vi "gen_logic_vi_with_cmd_array.vi"(9 "CmdInfo":T1, 10 "VI Paths":path) -> (2 "VI Paths Out":path=path "d:/Program Files (x86)/National Instruments/LabVIEW 2011/instr.lib/Agilent MXA Series/express/Utility/auto_gen_logic.vi")   [LabVIEW 2018]
uses:
  command_spec.ctl
  StudioHelper/Gtor/Mth/GenVI/Intf/GenStdVI/Mth/GenOneStdVI/TypeDefinitions/single_vi_spec.ctl
  StudioHelper/Gtor/Mth/GenVI/Intf/GenStdVI/Mth/GenOneStdVI/TypeDefinitions/single_cmd_spec.ctl
  StudioHelper/Gtor/Mth/GenVI/Intf/GenStdVI/Mth/GenOneStdVI/TypeDefinitions/single_control_spec.ctl
  StudioHelper/Gtor/Mth/GenVI/Intf/GenStdVI/Mth/GenOneStdVI/TypeDefinitions/control_data_type.ctl
  StudioHelper/Gtor/Mth/GenVI/Intf/GenStdVI/Mth/GenOneStdVI/TypeDefinitions/control_class.ctl
  StudioHelper/Gtor/Mth/GenVI/Intf/GenStdVI/Mth/GenOneStdVI/TypeDefinitions/ring_string_and_value.ctl
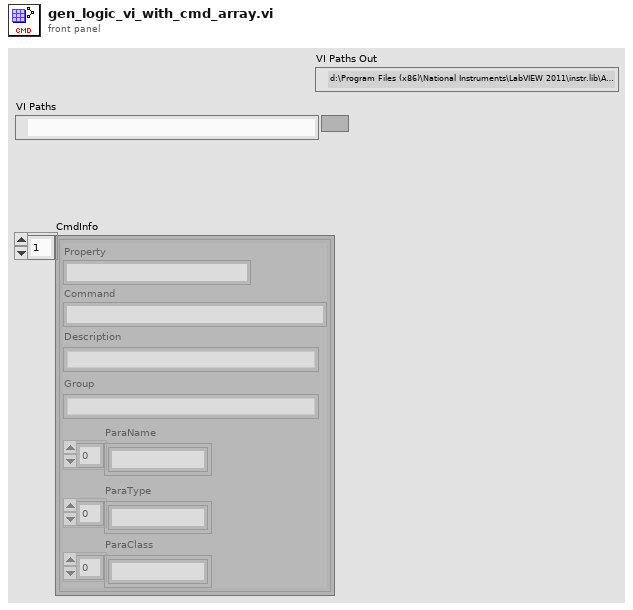
[diagram p1: front panel]
types:
  T1 = typedef "command_spec.ctl" = cluster{"Property":string, "Command":string, "Description":string, "Group":string, "ParaName":string[], "ParaType":string[], "ParaClass":string[]}[]
  T2 = typedef "single_vi_spec.ctl" = cluster{"Configure Specs In":T3[], "VI Paths":path, "Control Label Sequences":string[]}
  T3 = typedef "single_cmd_spec.ctl" = cluster{"Instrument Command":string, "Controls Specs":T4[]}
  T4 = typedef "single_control_spec.ctl" = cluster{"Control Label":string, "Control Data Type":T5, "Control Class":T6, "BD Text":string, "Ring Strings and Values":T7[], "Required Input":bool, "Default Value":string}
  T5 = typedef "control_data_type.ctl" = enum16{"DBL", "I32", "Boolean", "String", "U16", "U32", "EXT", "SGL", "I16", "U8", "I8", "I64", "U64", "Waveform", "Reference", "Variant", "Cluster"}
  T6 = typedef "control_class.ctl" = enum16{"Numeric", "Vertical Slide Switch", "Text Ring", "String", "Array", "VISAName", "WaveformGraph", "Cluster"}
  T7 = typedef "ring_string_and_value.ctl" = cluster{"String":string, "Value":dbl}
  T8 = typedef "auto_extracted_control_specs.ctl" = T9[]
  T9 = typedef "auto_extracted_control_spec.ctl" = cluster{"Control Data Type":T5, "Ring Text":string[], "Control Label":string, "Command Start Offset":i32, "Command Stop Offset":i32, "Control Class":T6, "Default Value":string, "Ring Strings and Values":T7[]}
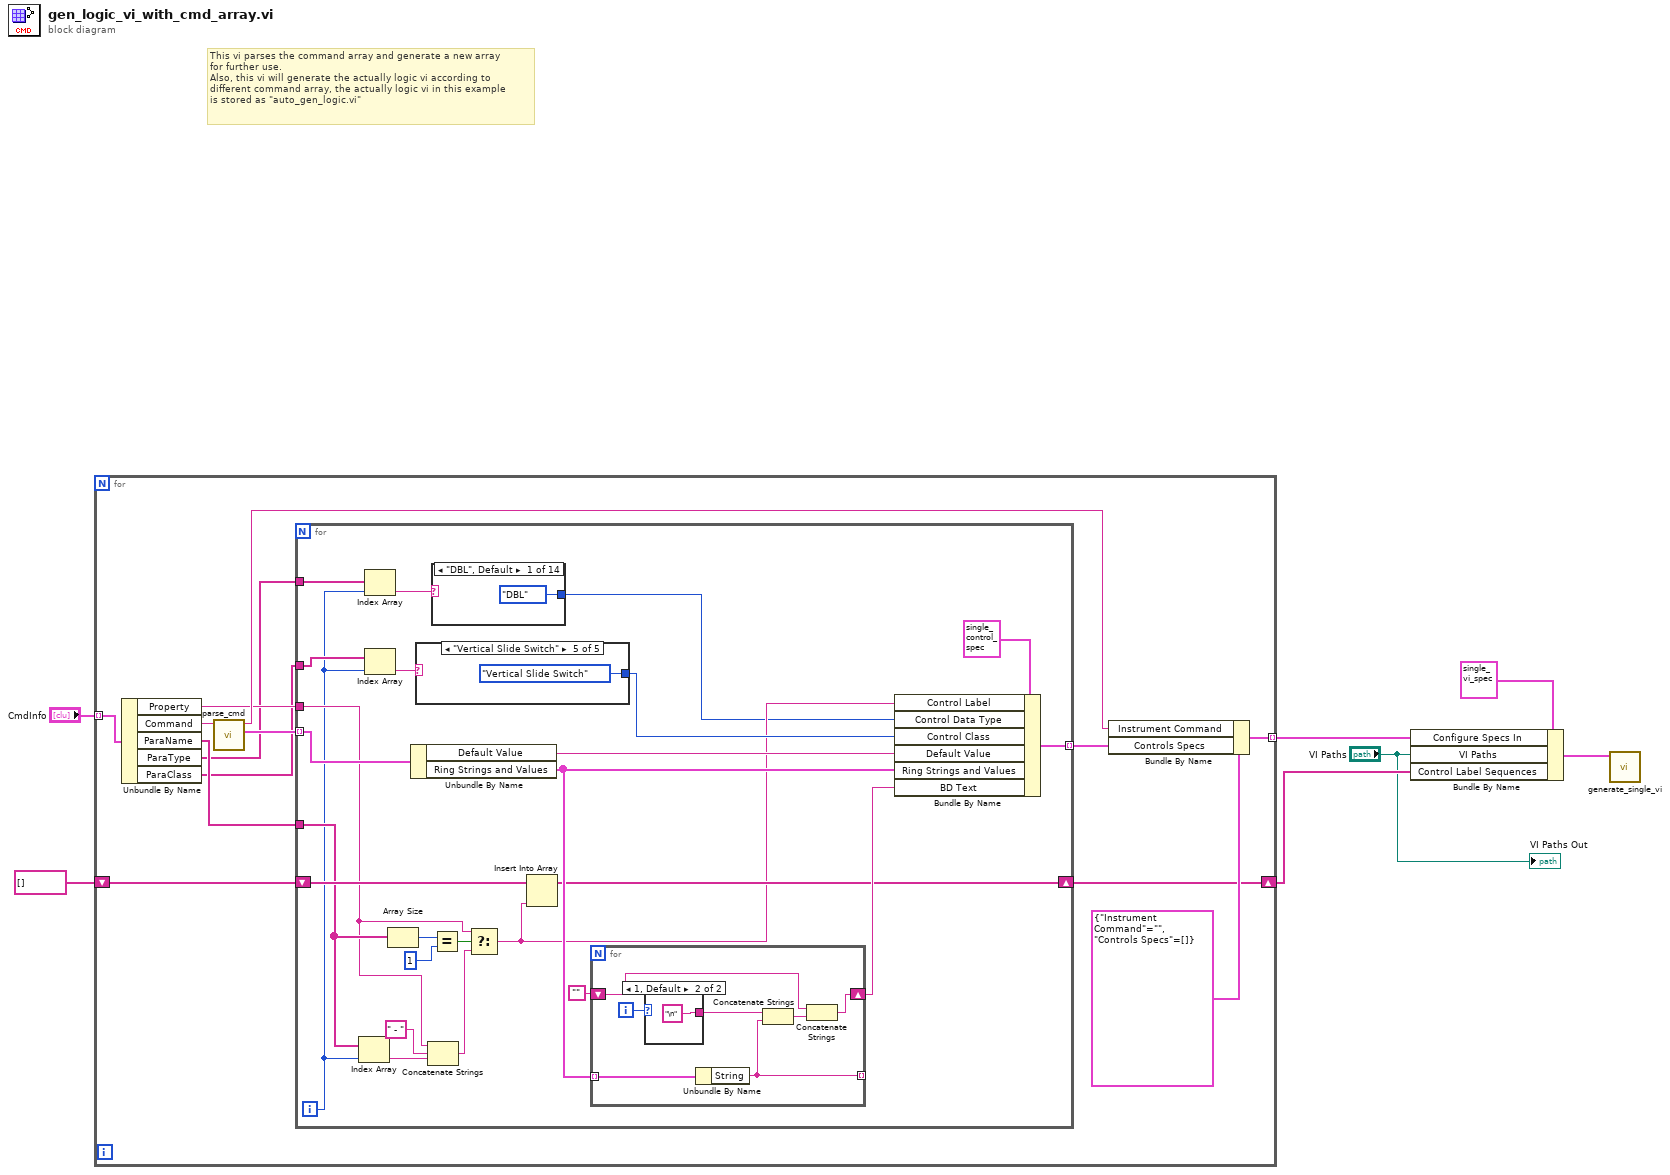
[diagram p0: block diagram]
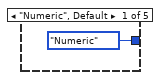
[diagram p2: hidden frame]
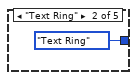
[diagram p3: hidden frame]
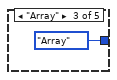
[diagram p4: hidden frame]
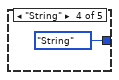
[diagram p5: hidden frame]
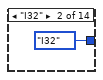
[diagram p6: hidden frame]
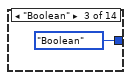
[diagram p7: hidden frame]
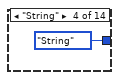
[diagram p8: hidden frame]
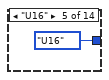
[diagram p9: hidden frame]
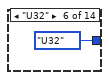
[diagram p10: hidden frame]
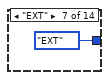
[diagram p11: hidden frame]
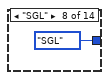
[diagram p12: hidden frame]
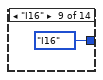
[diagram p13: hidden frame]
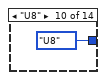
[diagram p14: hidden frame]
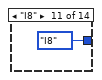
[diagram p15: hidden frame]
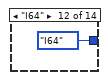
[diagram p16: hidden frame]
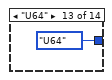
[diagram p17: hidden frame]
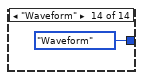
[diagram p18: hidden frame]
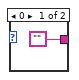
[diagram p19: hidden frame]
diagram:
  # "This vi parses the command array and generate a new array\nfor further use.\nAlso, this vi will generate the actually logic vi according to\ndifferent command array, the actually logic vi in this example\nis stored as \"auto_gen_logic.vi\""
  n1 = for {
    tunnel: [w18] -> w6 mode=indexing
    tunnel: "CmdInfo" -> [w17] mode=indexing
    shift-right: [w11] -> w3
    shift-left: string[] [] -> [w12]
    n2 = Unbundle By Name(w17) -> ("Property"=w15:string, "Command"=w16:string, "ParaName"=w10:string[], "ParaType"=w9:string[], "ParaClass"=w8:string[])
    n3 = call "parse_cmd.vi"("CMD In"=w16) -> ("CMD Parameters"=w13:T8, "CMD Out"=w19:string)  [unwired: 6 in, 3 out]
    n4 = for {
      tunnel: [w43] -> w14 mode=indexing
      tunnel: w15 -> [w29]
      tunnel: w13 -> [w39] mode=indexing
      shift-right: [w38] -> w11
      shift-left: w12 -> [w37]
      tunnel: w10 -> [w30]
      tunnel: w9 -> [w27]
      tunnel: w8 -> [w26]
      i -> [w25]
      n5 = Index Array(array=w30, index=w25) -> (element=w34:string)
      n6 = Index Array(array=w27, index=w25) -> (element=w23:string)
      n7 = Index Array(array=w26, index=w25) -> (element=w24:string)
      n8 = Array Size(array=w30) -> (size(s)=w31:i32)
      n9 = Unbundle By Name(w39) -> ("Default Value"=w44:string, "Ring Strings and Values"=w42:T7[])
      n10 = case shown="\"Vertical Slide Switch\"" w24 {
        tunnel: [control_class."Numeric" ("Control Class") control_class."Text Ring" ("Control Class") control_class."Array" ("Control Class") control_class."String" ("Control Class") control_class."Vertical Slide Switch" ("Control Class")] -> w28
        frame "Numeric", Default {
        }
        frame "Text Ring" {
        }
        frame "Array" {
        }
        frame "String" {
        }
        frame "Vertical Slide Switch" {
        }
      }
      n11 = Concatenate Strings(w29, " - " ("string"), w34) -> (w35:string)
      n12 = case shown="\"DBL\", Default" w23 {
        tunnel: [control_data_type."DBL" ("Control Data Type") control_data_type."I32" ("Control Data Type") control_data_type."Boolean" ("Control Data Type") control_data_type."String" ("Control Data Type") control_data_type."U16" ("Control Data Type") control_data_type."U32" ("Control Data Type") control_data_type."EXT" ("Control Data Type") control_data_type."SGL" ("Control Data Type") control_data_type."I16" ("Control Data Type") control_data_type."U8" ("Control Data Type") control_data_type."I8" ("Control Data Type") control_data_type."I64" ("Control Data Type") control_data_type."U64" ("Control Data Type") control_data_type."Waveform" ("Control Data Type")] -> w21
        frame "DBL", Default {
        }
        frame "I32" {
        }
        frame "Boolean" {
        }
        frame "String" {
        }
        frame "U16" {
        }
        frame "U32" {
        }
        frame "EXT" {
        }
        frame "SGL" {
        }
        frame "I16" {
        }
        frame "U8" {
        }
        frame "I8" {
        }
        frame "I64" {
        }
        frame "U64" {
        }
        frame "Waveform" {
        }
      }
      n13 = Equal?(x=w31, y=1) -> (x = y?=w36:bool)
      n14 = Select(t=w29, s=w36, f=w35) -> (s? t:f=w22:string)
      n15 = Insert Into Array(array=w37, new element=w22) -> (w38:string[])  [unwired: 1 in]
      n16 = for {
        tunnel: w42 -> [w71] mode=indexing
        shift-right: [w70] -> w40
        shift-left: "" -> [w69]
        tunnel: [w65] -> _ mode=indexing
        i -> [w66]
        n17 = case shown="1, Default" w66 {
          tunnel: ["" "\n" ("string")] -> w67
          frame 0 {
          }
          frame 1, Default {
          }
        }
        n18 = Unbundle By Name(w71) -> ("String"=w65:string)
        n19 = Concatenate Strings(w67, w65) -> (w68:string)
        n20 = Concatenate Strings(w69, w68) -> (w70:string)
      }
      n21 = Bundle By Name(cluster=T4 {"Control Label"="", "Control Data Type"=enum."DBL", "Control Class"=enum."Numeric", "BD Text"="", "Ring Strings and Values"=[], "Required Input"=FALSE, "Default Value"=""} ("Single Control Spec"), "Control Label"=w22, "Control Data Type"=w21, "Control Class"=w28, "Default Value"=w44, "Ring Strings and Values"=w42, "BD Text"=w40) -> (w43:T4)
    }
    n22 = Bundle By Name(cluster=T3 {"Instrument Command"="", "Controls Specs"=[]} ("Single Command Spec 2"), "Instrument Command"=w19, "Controls Specs"=w14) -> (w18:T3)
  }
  n23 = Bundle By Name(cluster=T2 {"Configure Specs In"=[{"Instrument Command"="%.;:CALC:MARK%s:PEAK:THR %g;", "Controls Specs"=[{"Control Label"="Ring0", "Control Data Type"=enum."I32", "Control Class"=enum."Text Ring", "BD Text"="1\n2\n3\n4\n5", "Ring Strings and Values"=[{"String"="1", "Value"=1.0}, {"String"="2", "Value"=2.0}, {"String"="3", "Value"=3.0}, {"String"="4", "Value"=4.0}, {"String"="5", "Value"=5.0}], "Required Input"=FALSE, "Default Value"=""}, {"Control Label"="<AMPL>", "Control Data Type"=enum."DBL", "Control Class"=enum."Numeric", "BD Text"="", "Ring Strings and Values"=[], "Required Input"=FALSE, "Default Value"=""}]}, {"Instrument Command"=":CALC:MARK%s:PEAK:TABL:READ %s;", "Controls Specs"=[{"Control Label"="Ring0", "Control Data Type"=enum."I32", "Control Class"=enum."Text Ring", "BD Text"="1\n2\n3\n4\n5", "Ring Strings and Values"=[{"String"="1", "Value"=1.0}, {"String"="2", "Value"=2.0}, {"String"="3", "Value"=3.0}, {"String"="4", "Value"=4.0}, {"String"="5", "Value"=5.0}], "Required Input"=FALSE, "Default Value"=""}, {"Control Label"="Ring2", "Control Data Type"=enum."I32", "Control Class"=enum."Text Ring", "BD Text"="ALL\rGTDL\rLTDL", "Ring Strings and Values"=[{"String"="ALL", "Value"=0.0}, {"String"="LTDL", "Value"=2.0}], "Required Input"=FALSE, "Default Value"=""}]}, {"Instrument Command"=":CALC:MARK:TABL %d,%s;", "Controls Specs"=[{"Control Label"="int0", "Control Data Type"=enum."I32", "Control Class"=enum."Numeric", "BD Text"="", "Ring Strings and Values"=[], "Required Input"=FALSE, "Default Value"=""}, {"Control Label"="Bool0", "Control Data Type"=enum."Boolean", "Control Class"=enum."Vertical Slide Switch", "BD Text"="", "Ring Strings and Values"=[], "Required Input"=FALSE, "Default Value"=""}]}], "VI Paths"=path "", "Control Label Sequences"=[]} ("Single VI Spec"), "Configure Specs In"=w6, "VI Paths"="VI Paths", "Control Label Sequences"=w3) -> (w1:T2)
  n24 = call "generate_single_vi.vi"("Single VI Spec"=w1) -> ()  [unwired: 10 in, 1 out]
  "VI Paths Out" <- "VI Paths"
